vi "subDFD_Extract String between Tags.vi"(7 "whitespace location":T1=2 items=["both", "start of string", "end of string"], 9 "tag":string, 10 "original string":string) -> (2 "extracted string":string)   [LabVIEW 2023]
uses:
  <vilib>/Utility/error.llb/whitespace.ctl
  <vilib>/Utility/error.llb/Trim Whitespace One-Sided.vi
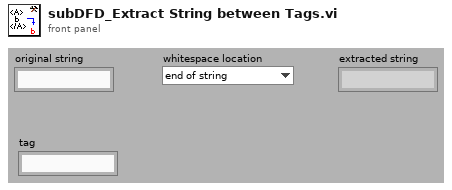
[diagram p1: front panel]
types:
  T1 = typedef "whitespace.ctl" = u16
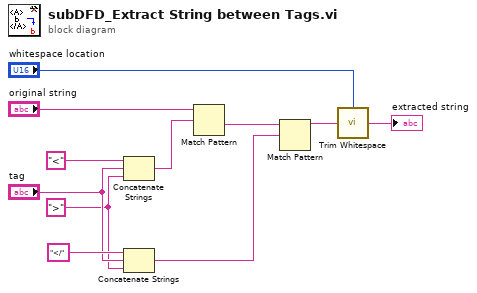
[diagram p0: block diagram]
diagram:
  w4 = ">"
  n1 = Concatenate Strings("<", "tag", w4) -> (w9:string)
  n2 = Concatenate Strings("</", "tag", w4) -> (w10:string)
  n3 = Match Pattern(string="original string", regular expression=w9) -> (after substring=w11:string)  [unwired: 4 out]
  n4 = Match Pattern(string=w11, regular expression=w10) -> (before substring=w3:string)  [unwired: 4 out]
  n5 = call <vilib>:"Trim Whitespace.vi"("string"=w3, "location (both)"="whitespace location") -> ("trimmed string"=→"extracted string":string)
